vi "TLB Native Dynamic Events ver 0.11.vi"() -> ()   [LabVIEW 2018]
uses:
  Labview Training Phase 2/Enum Controls/States for Action Engine.ctl
  TLB Type Definitions/State Type Definitions, for 0.26g versions and later 2.ctl
  TLB Type Definitions/Intruction Type Definitions.ctl
  TLB Type Definitions/Encoder cluster.ctl
  Experimental VI's/Archived VI's/MOTOR CONTROL NO PID Type Def.ctl
  Underlying VI's/I2C Master VI/I2C MASTER Type Def.ctl
  TLB Type Definitions/PING CLUSTER.ctl
  <vilib>/Studica/Studica Toolkit/NavX/NavX.lvlib
  <vilib>/Studica/Studica Toolkit/Background/DIO Channel.ctl
  Underlying VI's/NavX VI/navX type def.ctl
  <vilib>/myRIO/Instrument Drivers/Utilities/Utilities.lvlib
  <vilib>/Studica/Studica Toolkit/Background/I2C Channel.ctl
  <vilib>/Studica/Studica Toolkit/NavX/TypeDefs/Flags/Z900_navX_Flags_CalibrationStatusTypeDef.ctl
  <vilib>/Studica/Studica Toolkit/NavX/TypeDefs/Flags/Z900_navX_Flags_OpStatusTypeDef.ctl
panel:
  out "Detect?":bool
  out "Status":T3 {"OP Status" items=["INITIALIZING", "SELFTEST_IN_PROGRESS", "ERROR", "IMU_AUTOCAL_IN_PROGRESS", "NORMAL"]; "Calibration Status" items=["IMU_CAL_STATE_MASK"=3, "IMU_CAL_STATE_INPROGRESS"=0, "IMU_CAL_STATE_ACCUMULATE"=1, "IMU_CAL_STATE_COMPLETE"=2]}
  out "NavX Readings":T4
  out "TASK ENABLE":bool
  out "Rising Edge":bool
  in  "Green LED":bool
  out "Task Selection":u8
  out "Object detected?":bool
  in  "Arduino Mode":T5=enum."Mode 0"
  out "Arduino Data":T6
  out "I2C Error":errorcluster
  out "Speed & distance":T7
  out "State Logic":T8=enum."Startup"
  out "elements":T9[](array[typedef])
  in  "STOP TASK":bool
  in  "OK Button":bool
  in  "STOP":bool
  out "error out":errorcluster
  out "Action Queue Items":i32
  out "State Logic Queue Items":i32
  out "Action Queues items":string[](array[string])=["Hardware reset", "Software reset", ""]
  out "Action State":string
  # "TLB FRAMEWORK STATUS"
  # "System Health Status Update"
  # "Test Programme written by Calvin Loke    Dated: 28 Aug 2019\nTest Programme revised by Dr Alex See   Dated 30 Aug 2019\n\nProgramme version:   TLB Native Dynamic Events ver 0.04b.vi"
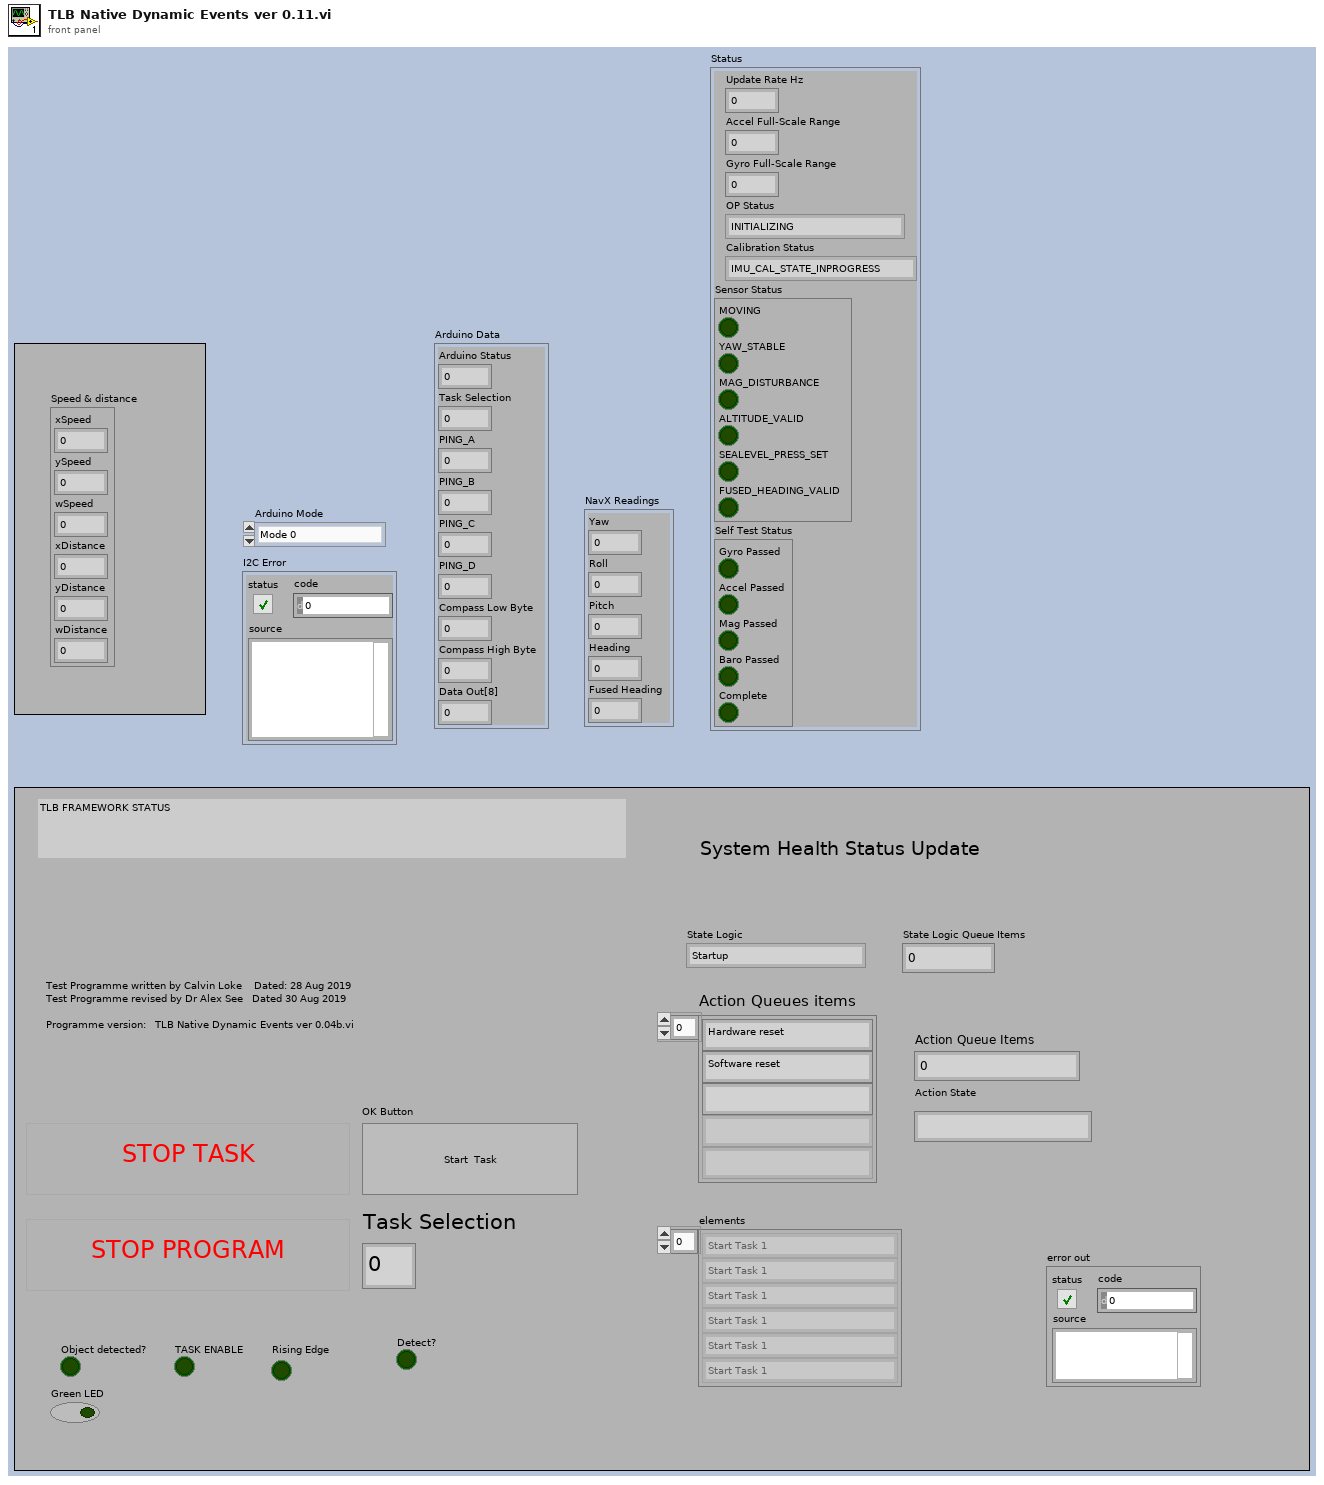
[diagram p1: front panel]
types:
  T1 = typedef "NavX.lvlib/Z900_navX_Flags_OpStatusTypeDef.ctl" = u8
  T2 = typedef "NavX.lvlib/Z900_navX_Flags_CalibrationStatusTypeDef.ctl" = u8
  T3 = cluster{"Update Rate Hz":u8, "Accel Full-Scale Range":u8, "Gyro Full-Scale Range":u16, "OP Status":T1, "Calibration Status":T2, "Sensor Status":cluster{"MOVING":bool, "YAW_STABLE":bool, "MAG_DISTURBANCE":bool, "ALTITUDE_VALID":bool, "SEALEVEL_PRESS_SET":bool, "FUSED_HEADING_VALID":bool}, "Self Test Status":cluster{"Gyro Passed":bool, "Accel Passed":bool, "Mag Passed":bool, "Baro Passed":bool, "Complete":bool}}
  T4 = cluster{"Yaw":dbl, "Roll":dbl, "Pitch":dbl, "Heading":dbl, "Fused Heading":dbl}
  T5 = typedef "I2C MASTER Type Def.ctl" = enum16{"Last State", "Mode 0", "Mode 1", "Mode 2", "Mode 3", "Mode 4", "Mode 5", "Mode 6", "Mode 7", "Mode 8", "Mode 9", "Mode 10"}
  T6 = cluster{"Arduino Status":u8, "Task Selection":u8, "PING_A":u8, "PING_B":u8, "PING_C":u8, "PING_D":u8, "Compass Low Byte":u8, "Compass High Byte":u8, "Data Out[8]":u8}
  T7 = cluster{"xSpeed":dbl, "ySpeed":dbl, "wSpeed":dbl, "xDistance":dbl, "yDistance":dbl, "wDistance":dbl}
  T8 = typedef "State Type Definitions, for 0.26g versions and later 2.ctl" = enum16{"None", "Startup", "Move to Angle", "True Stop", "Idle", "Shutdown", "Task 1A", "Task 1B", "Task 2:Raise Arm", "Task 2:Sensor Mode", "Task 2:Reverse Mode", "Task 3", "Task 4_A", "Task 4_B", "Task 4_C", "Task 4_D", "Task 5A", "Task 5B", "Task 5C", "Task 5D", "Task 5E: POSITION ARM", "Task 5F: ARM GRAB HEIGHT", "Task 5G: CLOSE CLAW", "Task 5H: RAISE ARM", "Task 6_A", "Task 6_B", "Task 7", "Task 8A: RAISE ARM", "Task 8B: MOVE TO BOX", "Task 8C: CAM BURST", "Task 8D: PROCESS IMAGE", "Task 8E: ROBOT ADJUST", "Task 8F: CAM BURST 2", "Task 8G: PROCESS IMAGE 2", "Task 8H: ARM ADJUST", "Task 8I: ARM GRAB HEIGHT", "Task 8J: CLOSE CLAW", "Task 8K: RAISE MY SWORD", "Task 9A: Raise Arm", "Task 9B: Rotate to Angle", "Task 9C: Detect Box", "Task 9D: MOVE FORWARD", "Task 9E: MOVE LEFT", "Task 9F: SCAN BOX", "Task 9G: MOVE RIGHT", "Task 9H: SCAN BOX 2", "Task 9I: ROTATE 90 CW", "Task 9J: FORWARD", "Task 9K: RAM WALL", "Task 9L: MOVE RIGHT", "Task 9M: SCAN BOX 3", "Task 9M: MOVE RIGHT", "Task 9N: SCAN BOX 4", "PENIS", "PENIS 2", "PENIS 3", "Task 9R: PROCESS COLOUR", "Task A1: Task 9 Open cam", "Task A2: Task 9 Move Arm", "Task A3: Task 9 Set Timer", "Task A4: Tasl 9 Capture images", "Task A5: Task 9 Close camera", "Task A6: Process Colour", "Task A7: Dispose Camera Buffer"}
  T9 = typedef "Intruction Type Definitions.ctl" = enum16{"None", "Start Task 1", "Start Task 2", "Start Task 3", "Start Task 4", "Start Task 5", "Start Task 6", "Start Task 7", "Start Task 8 - BALL", "Start Task 8 - Gel", "Start Task 8 - Pipe", "Start Task 8 - Soap", "Start Task 9", "Start Task A", "Start Task B", "Exit"}
  T10 = typedef "States for Action Engine.ctl" = enum16{"Initialize", "Write", "Read"}
  T11 = typedef "DIO Channel.ctl" = enum16{"Not Connected", "A/DIO1", "A/DIO2", "A/DIO3", "A/DIO4", "A/DIO5", "A/DIO6", "A/DIO7", "A/DIO13", "B/DIO1", "B/DIO2", "B/DIO3", "B/DIO4", "B/DIO5", "B/DIO6", "B/DIO7", "B/DIO13", "C/DIO0", "C/DIO1", "C/DIO2", "C/DIO3", "C/DIO4", "C/DIO5", "C/DIO6", "C/DIO7"}
  T12 = typedef "PING CLUSTER.ctl" = cluster{"PING_A":u8, "PING_B":u8, "PING_C":u8, "PING_D":u8}
  T13 = typedef "Encoder cluster.ctl" = cluster{"xDistance":dbl, "yDistance":dbl, "wDistance":dbl}
  T14 = typedef "I2C Channel.ctl" = enum16{"Not Connected", "A", "B"}
  T15 = typedef "navX type def.ctl" = enum16{"Get i2C reference", "Read Values", "Zero Yaw"}
  T16 = typedef "State Type Definitions.ctl" = enum16{"None", "Startup", "Move to Angle", "True Stop", "Idle", "Shutdown", "Task 1", "Task 2:Raise Arm", "Task 2:Sensor Mode", "Task 2:Reverse Mode", "Task 3", "Task 4_A", "Task 4_B", "Task 4_C", "Task 4_D", "Task 5A: ARM CAM HEIGHT", "Task 5B: MOVE TO BOX", "Task 5C: CAM BURST", "Task 5D: PROCESS IMAGE", "Task 5E: POSITION ARM", "Task 5F: ARM GRAB HEIGHT", "Task 5G: CLOSE CLAW", "Task 5H: RAISE ARM", "Task 6_A", "Task 6_B", "Task 7", "Task 8A: RAISE ARM", "Task 8B: MOVE TO BOX", "Task 8C: CAM BURST", "Task 8D: PROCESS IMAGE", "Task 8E: ROBOT ADJUST", "Task 8F: CAM BURST 2", "Task 8G: PROCESS IMAGE 2", "Task 8H: ARM ADJUST", "Task 8I: ARM GRAB HEIGHT", "Task 8J: CLOSE CLAW", "Task 8K: RAISE MY SWORD", "Task 9A: Raise Arm", "Task 9B: Rotate to Angle", "Task 9C: Detect Box", "Task 9D: MOVE FORWARD", "Task 9E: MOVE LEFT", "Task 9F: SCAN IMAGE", "Task 9G: PROCESS COLOUR", "Task 9H: MOVE RIGHT", "Task 9I: SCAN IMAGE", "Task 9J: PROCESS COLOUR", "Task 9K: ROTATE 90 CW", "Task 9L: MOVE FORWARD", "Task 9M: MOVE RIGHT", "Task 9N: SCAN IMAGE", "Task 9O: PROCESS COLOUR", "Task 9P: MOVE RIGHT", "Task 9Q: SCAN IMAGE", "Task 9R: PROCESS COLOUR"}
  T17 = typedef "State Type Definitions.ctl" = enum16{"None", "Startup", "Move to Angle", "True Stop", "Idle", "Shutdown", "Task 1", "Task 2", "Task 3", "Task 4_A", "Task 4_B", "Task 4_C", "Task 5", "Task 6", "Task 7", "Task 8", "Task 9", "Task A", "Task B"}
  T18 = typedef "MOTOR CONTROL NO PID Type Def.ctl" = enum16{"Init", "Front Back", "Left Right", "Rotate", "Stop", "Latch"}
  T19 = cluster{"DIO Channel":T11, "FPGA VI Reference Out":refnum<k20>}
  T20 = cluster{"I2C Ref Out":cluster{"I2C Channel":T14, "FPGA VI Reference Out":refnum<k20>}, "Connected":bool, "Slave Address (7-bit)":u8, "Registry":u8[]}
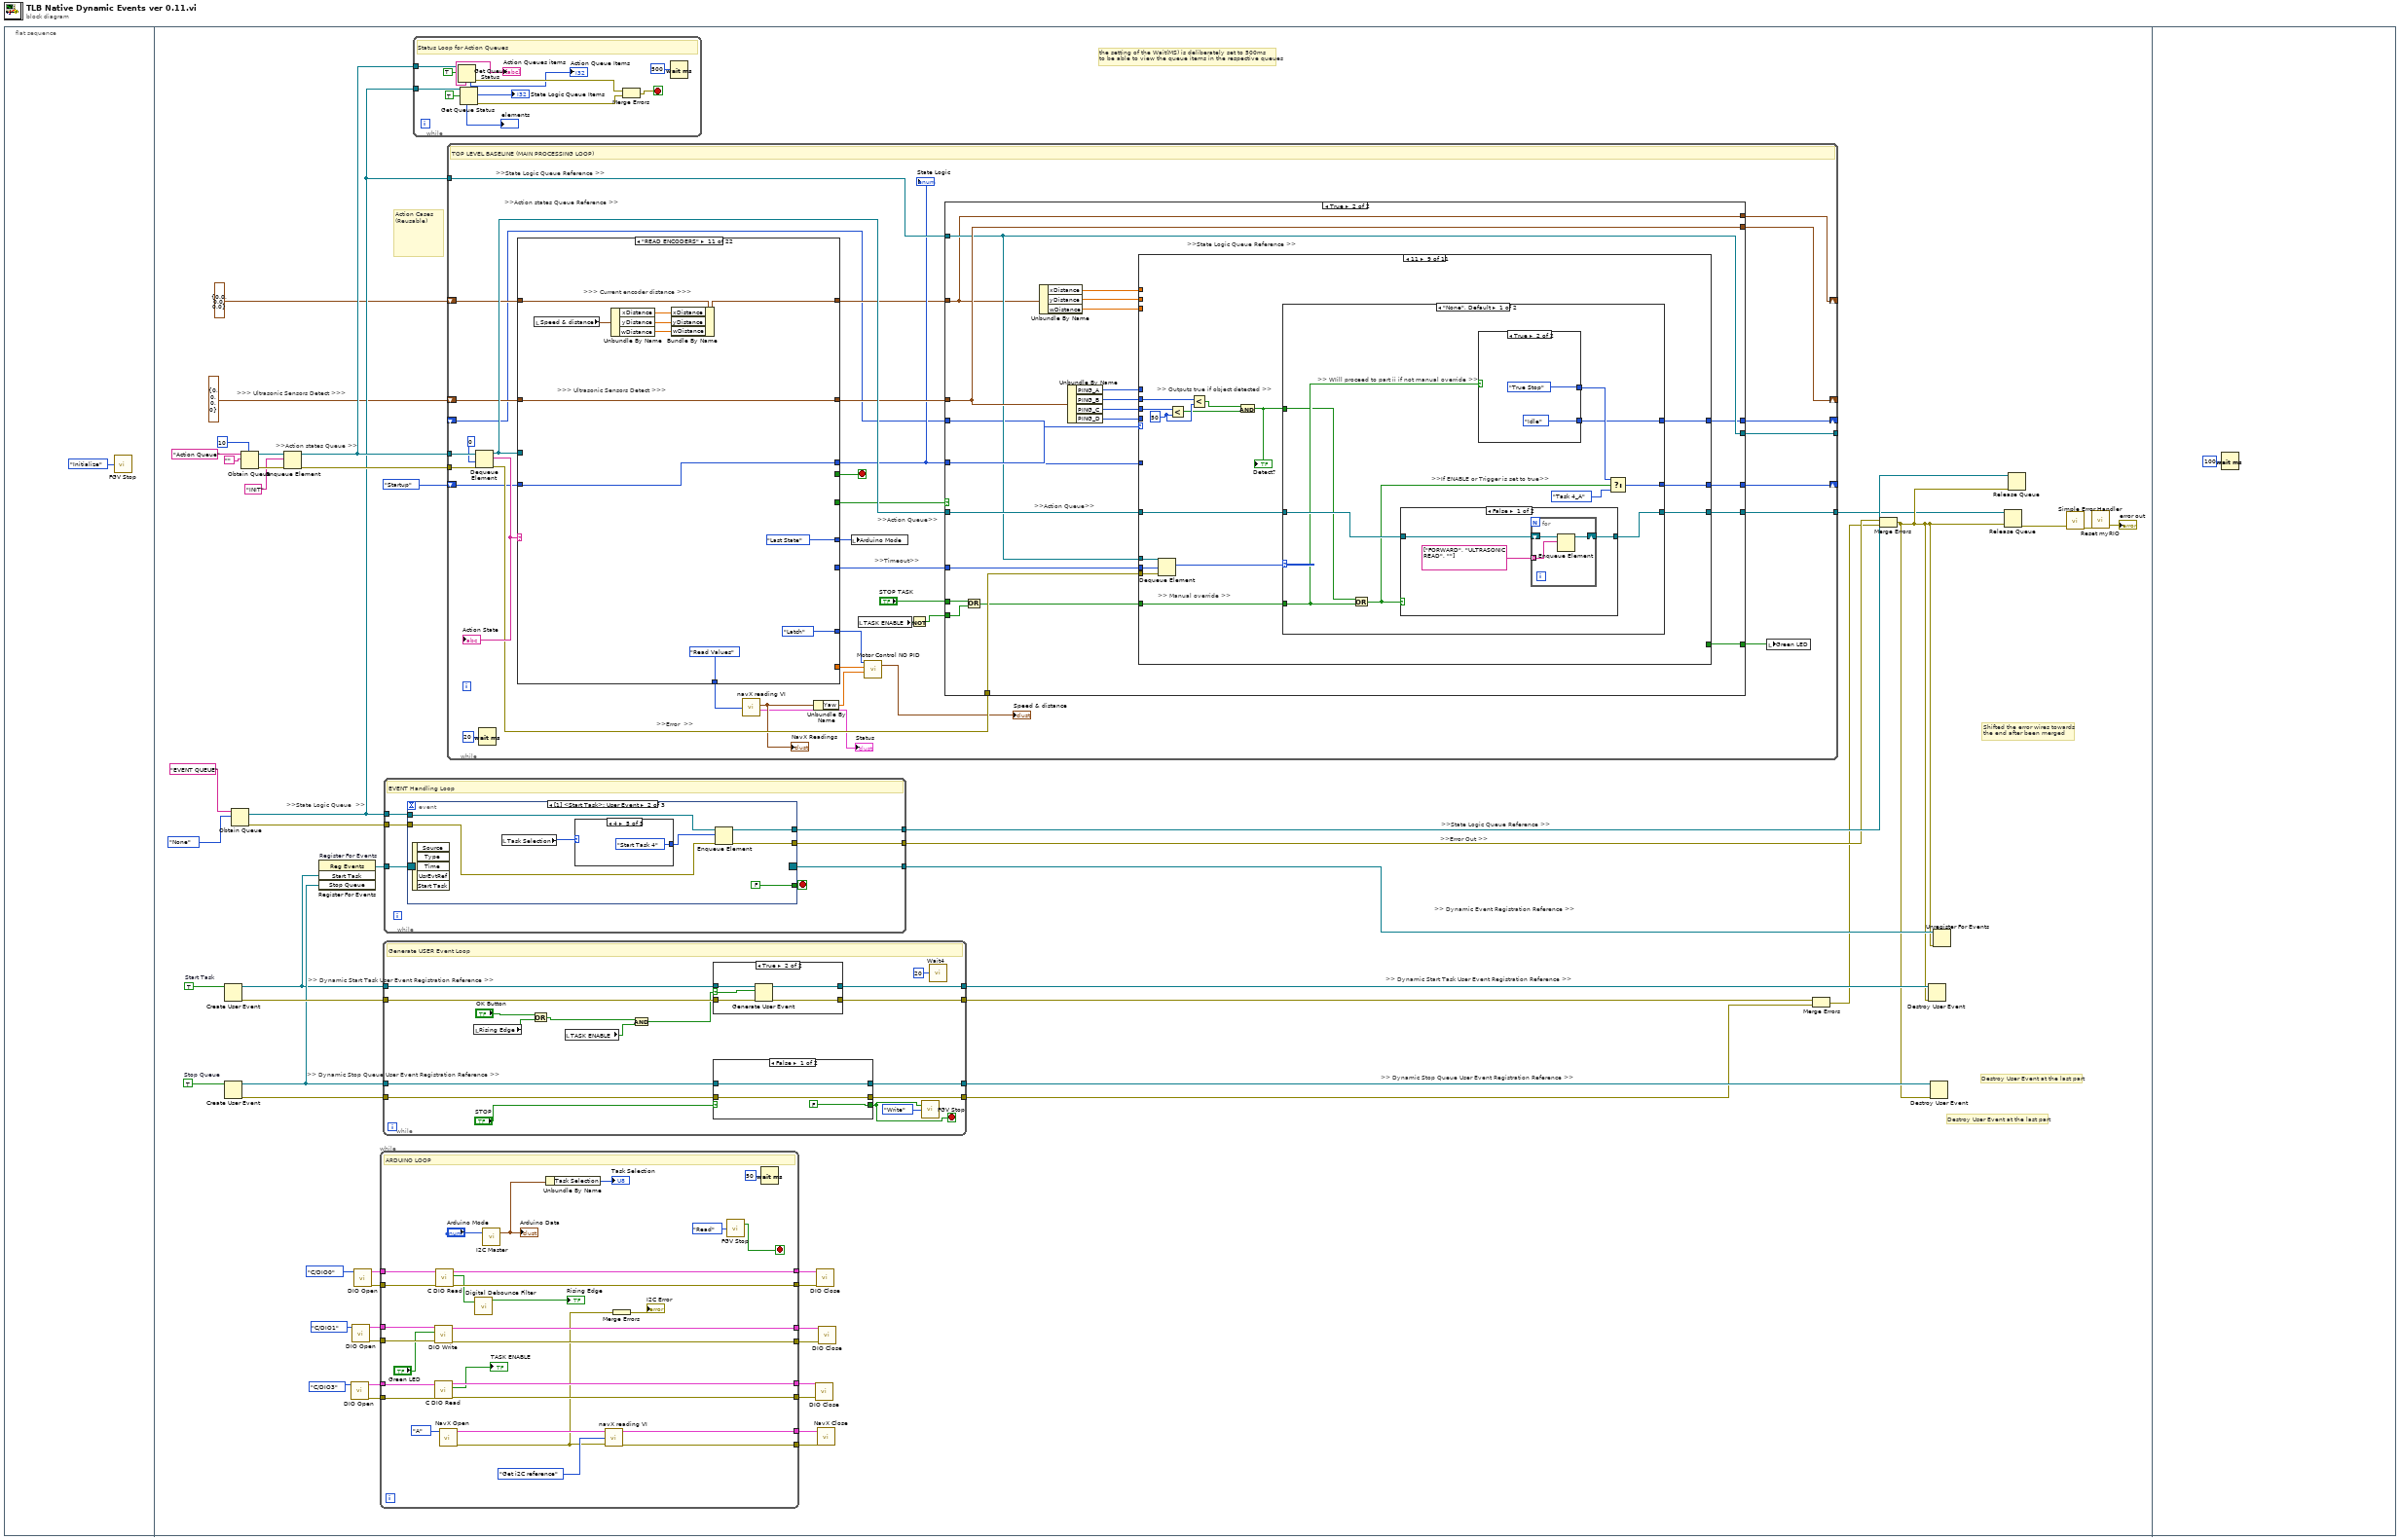
[diagram p0: block diagram]
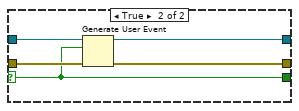
[diagram p2: hidden frame]
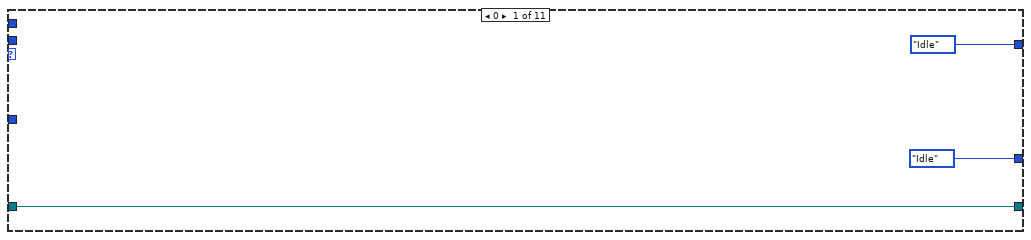
[diagram p5: hidden frame]
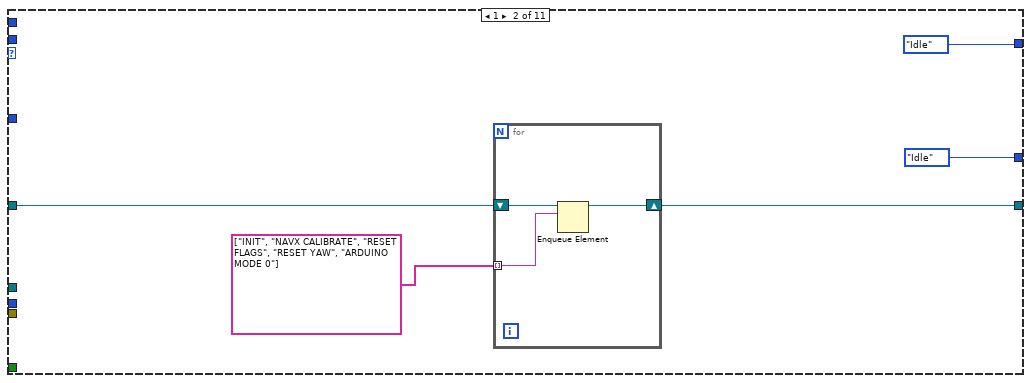
[diagram p6: hidden frame]
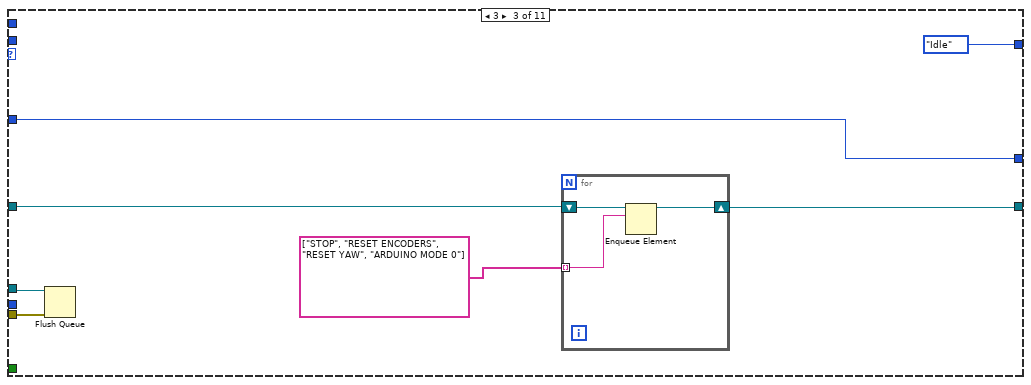
[diagram p7: hidden frame]
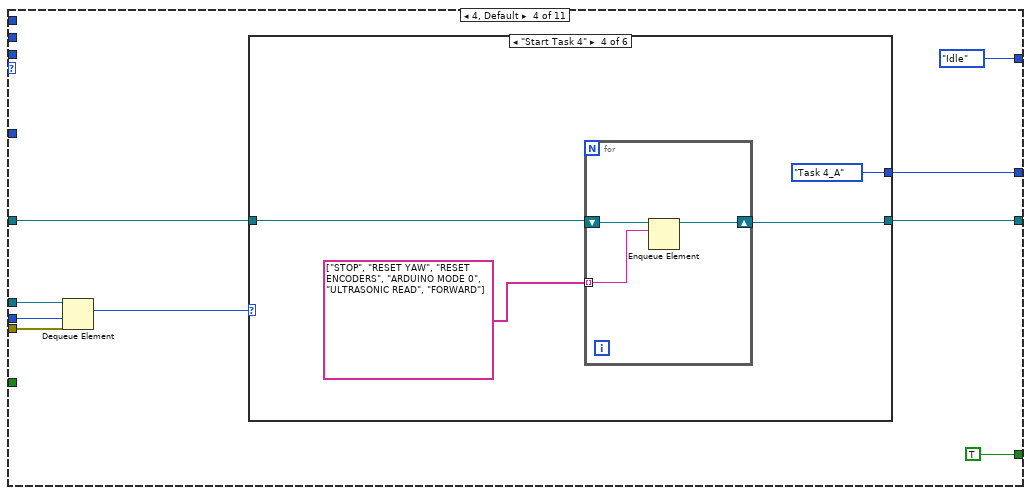
[diagram p8: hidden frame]
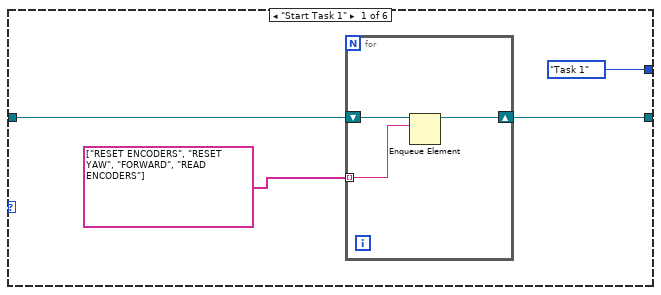
[diagram p9: hidden frame]
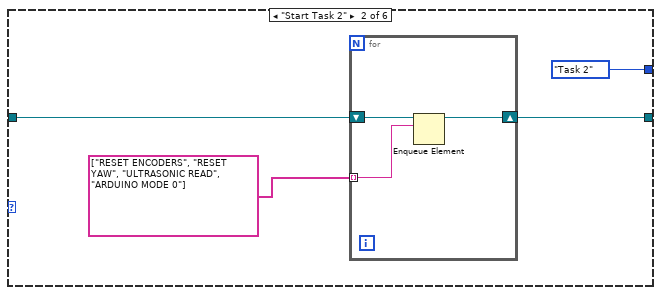
[diagram p10: hidden frame]
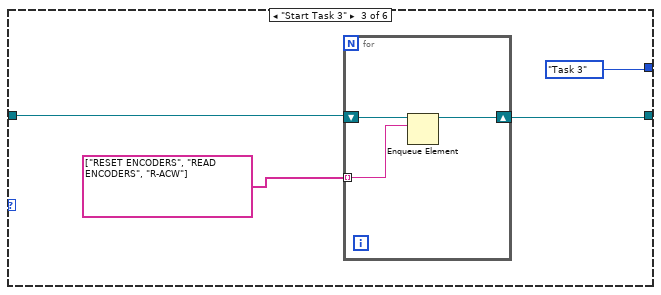
[diagram p11: hidden frame]
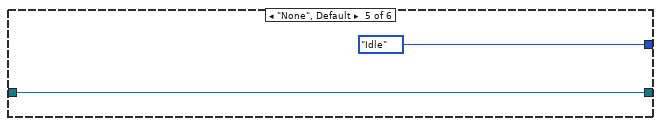
[diagram p12: hidden frame]
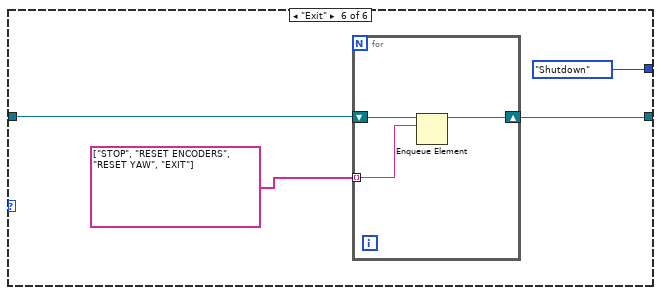
[diagram p13: hidden frame]
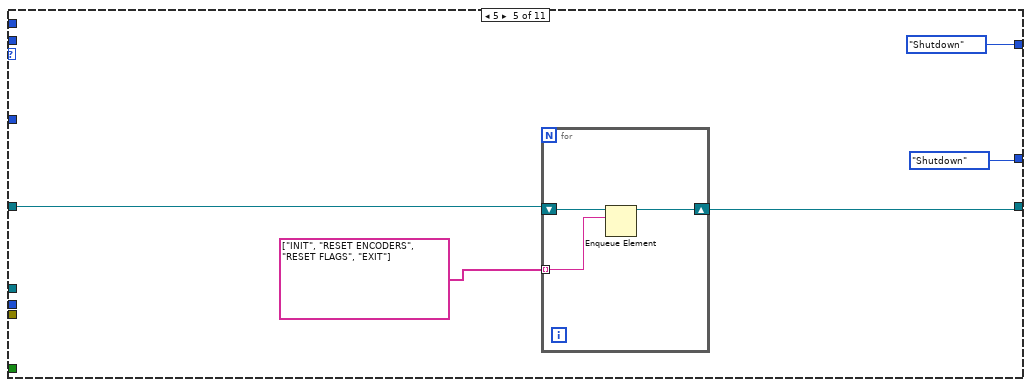
[diagram p14: hidden frame]
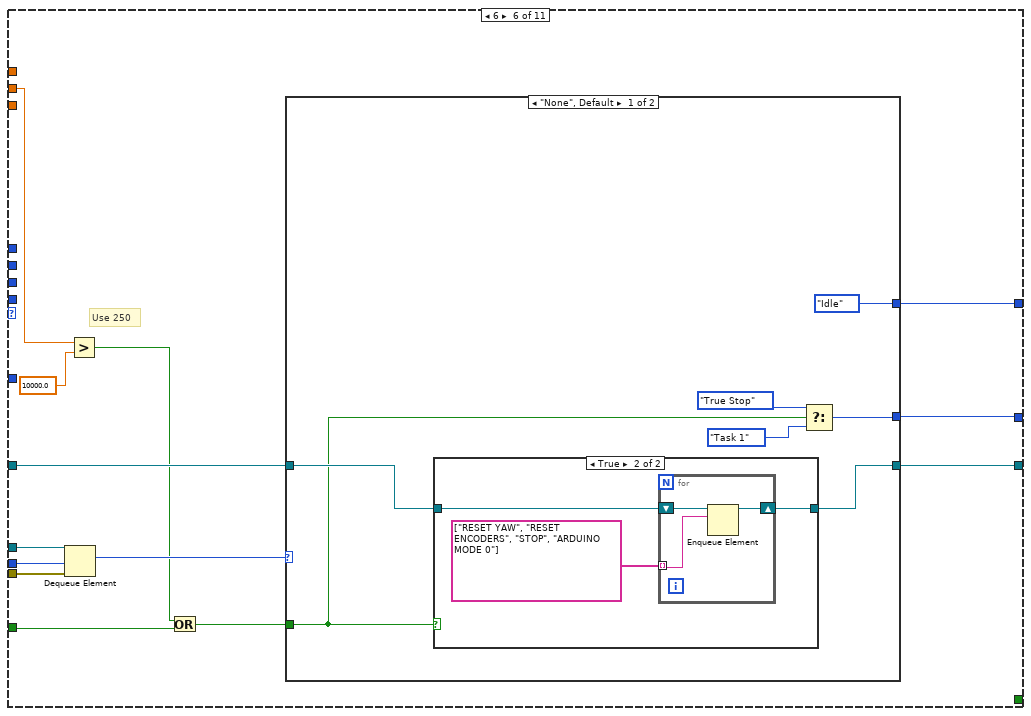
[diagram p15: hidden frame]
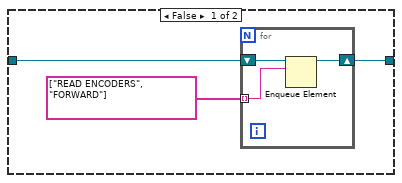
[diagram p16: hidden frame]
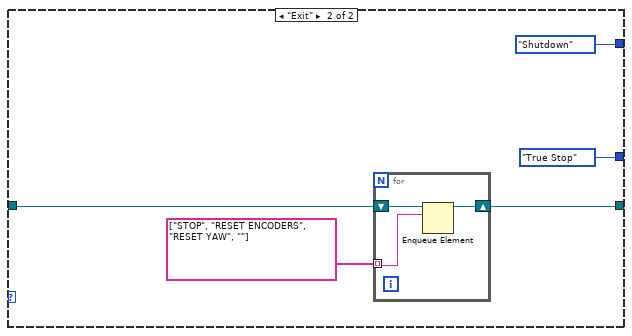
[diagram p17: hidden frame]
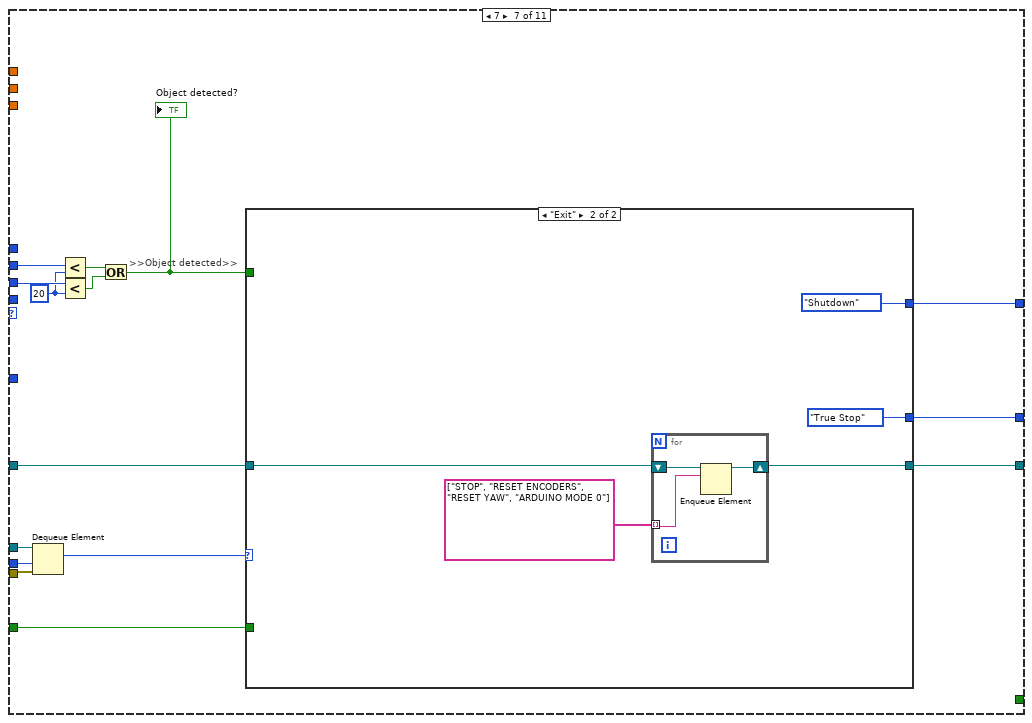
[diagram p18: hidden frame]
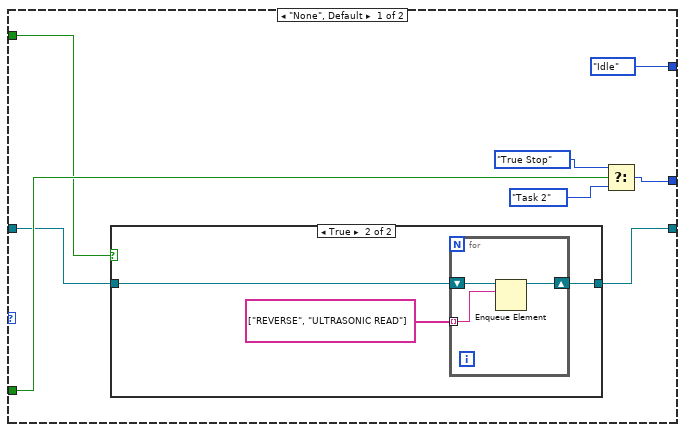
[diagram p19: hidden frame]
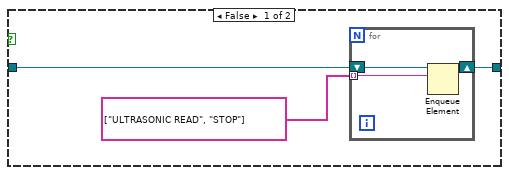
[diagram p20: hidden frame]
diagram:
  n1 = flat-sequence {
    frame #0 {
      n2 = call "FGV Stop.vi"("Init/Read/Write State"=States_for_Action_Engine."Initialize") -> ()  [unwired: 2 in, 2 out]
    }
    frame #1 {
      w53 = TRUE  # Stop Queue
      w52 = TRUE  # Start Task
      # ">>> Ultrasonic Sensors Detect >>>"
      # "the setting of the Wait(MS) is deliberately set to 500ms\nto be able to view the queue items in the respective queues"
      # "Action Cases\n(Reusable)"
      # ">>Error Out >>"
      # ">> Dynamic Stop Queue User Event Registration Reference >>"
      # ">> Dynamic Start Task User Event Registration Reference >>"
      # ">> Dynamic Stop Queue User Event Registration Reference >>"
      # ">> Dynamic Start Task User Event Registration Reference >>"
      # ">> Dynamic Event Registration Reference >>"
      # ">>Action states Queue >>"
      # ">>State Logic Queue  >>"
      # ">>State Logic Queue Reference >>"
      # "Destroy User Event at the last part"
      # "Destroy User Event at the last part"
      # "Shifted the error wires towards\nthe end after been merged"
      n3 = Create User Event(user event datatype=w52) -> (user event=w44:refnum<user-event>, error out=w49:errorcluster)  [unwired: 1 in]
      n4 = Create User Event(user event datatype=w53) -> (user event=w45:refnum<user-event>, error out=w48:errorcluster)  [unwired: 1 in]
      n5 = Obtain Queue(name (unnamed)="EVENT QUEUE", element data type=Intruction_Type_Definitions."None" ("Enum")) -> (queue out=w30:refnum<queue>, error out=w36:errorcluster)  [unwired: 3 in, 1 out]
      n6 = Obtain Queue(max queue size (-1, unlimited)=10, name (unnamed)="Action Queue", element data type="") -> (queue out=w39:refnum<queue>, error out=w35:errorcluster)  [unwired: 2 in, 1 out]
      n7 = Enqueue Element(queue=w39, element="INIT", error in (no error)=w35) -> (queue out=w31:refnum<queue>, error out=w34:errorcluster)  [unwired: 1 in, 1 out]
      n8 = register-events "Register For Events"(w44, w45) -> (reference out=w43:refnum<event-registration>)  [unwired: 2 in, 1 out]
      n9 = call <vilib>:"DIO Open.vi"("DIO Channel"=DIO_Channel."C/DIO3") -> ("error out"=w8:errorcluster, "DIO Info Out"=w9:T19)  [unwired: 9 in]
      n10 = call <vilib>:"DIO Open.vi"("DIO Channel"=DIO_Channel."C/DIO1") -> ("error out"=w13:errorcluster, "DIO Info Out"=w15:T19)  [unwired: 9 in]
      n11 = call <vilib>:"DIO Open.vi"("DIO Channel"=DIO_Channel."C/DIO0") -> ("error out"=w18:errorcluster, "DIO Info Out"=w21:T19)  [unwired: 9 in]
      n12 = while {
        tunnel: w21 -> [w77]
        tunnel: [w76] -> w19
        tunnel: w18 -> [w75]
        tunnel: [w74] -> w17
        tunnel: w15 -> [w69]
        tunnel: [w68] -> w14
        tunnel: w13 -> [w67]
        tunnel: [w66] -> w12
        tunnel: [w64] -> w10
        tunnel: w9 -> [w63]
        tunnel: w8 -> [w62]
        tunnel: [w61] -> w7
        tunnel: [w58] -> w6
        tunnel: [w57] -> w5
        stop <- w81 stop-if-true
        # "ARDUINO LOOP"
        n13 = call <vilib>:"DIO Write.vi"("error in (no error)"=w67, "Input"="Green LED", "DIO Info In"=w69) -> ("error out"=w66:errorcluster, "DIO Info Out"=w68:T19)  [unwired: 7 in]
        n14 = call <vilib>:"C DIO Read.vi"("error in (no error)"=w62, "DIO Info In in"=w63) -> ("error out"=w61:errorcluster, "IN"=→"TASK ENABLE":bool, "DIO Info In out"=w64:T19)  [unwired: 7 in]
        n15 = call <vilib>:"C DIO Read.vi"("error in (no error)"=w75, "DIO Info In in"=w77) -> ("error out"=w74:errorcluster, "IN"=w72:bool, "DIO Info In out"=w76:T19)  [unwired: 7 in]
        n16 = call <vilib>:"NavX Open.vi"("I2C Channel"=I2C_Channel."A") -> ("error out"=w55:errorcluster, "NavX Info"=w59:T20)  [unwired: 9 in]
        n17 = call "Digital Debounce Filter.vi"("Boolean input"=w72) -> ("Rising Edge"=→"Rising Edge":bool)  [unwired: 1 in, 2 out]
        n18 = call "I2C Master.vi"("Arduino Mode"="Arduino Mode") -> ("Arduino Data"=w70:T6)  [unwired: 1 in, 1 out]
        "Arduino Data" <- w70
        n19 = Unbundle By Name(w70) -> ("Task Selection"=→"Task Selection":u8)
        n20 = call "navX reading VI.vi"("NavX Info In"=w59, "Mode"=navX_type_def."Get i2C reference", "error in (no error)"=w55) -> ("NavX Info Out"=w58:T20, "Error Out"=w57:errorcluster)  [unwired: 2 out]
        n21 = Merge Errors(w55) -> (→"I2C Error":errorcluster)
        n22 = call "FGV Stop.vi"("Init/Read/Write State"=States_for_Action_Engine."Read") -> ("Output node"=w81:bool)  [unwired: 2 in, 1 out]
        n23 = Wait (ms)(milliseconds to wait=u32 50) -> ()  [unwired: 1 out]
      }
      n24 = while {
        tunnel: w44 -> [w111]
        tunnel: w45 -> [w110]
        tunnel: [w109] -> w51
        tunnel: [w108] -> w50
        tunnel: w49 -> [w107]
        tunnel: [w106] -> w47
        tunnel: w48 -> [w105]
        tunnel: [w104] -> w46
        stop <- w102 stop-if-true
        # "Generate USER Event Loop"
        n25 = local read "Rising Edge"() -> (w98:bool)
        n26 = Or(x="OK Button", y=w98) -> (x .or. y?=w97:bool)
        n27 = local read "TASK ENABLE"() -> (w96:bool)
        n28 = And(x=w97, y=w96) -> (x .and. y?=w95:bool)
        n29 = case shown="True" w95 {
          selector: w95 -> [_ w122]
          tunnel: w111 -> [w121 w126]
          tunnel: [w121 w125] -> w108
          tunnel: w107 -> [w120 w124]
          tunnel: [w120 w123] -> w106
          frame False {
          }
          frame True {
            n30 = Generate User Event(user event=w126, event data cluster=w122, error in=w124) -> (user event out=w125:refnum<user-event>, error out=w123:errorcluster)  [unwired: 1 in]
          }
        }
        n31 = case shown="False" "STOP" {
          selector: "STOP" -> [_ w115]
          tunnel: w110 -> [w114 w119]
          tunnel: [w114 w118] -> w109
          tunnel: w105 -> [w113 w117]
          tunnel: [w113 w116] -> w104
          tunnel: [FALSE w115] -> w102
          frame False {
          }
          frame True {
            n32 = Generate User Event(user event=w119, event data cluster=w115, error in=w117) -> (user event out=w118:refnum<user-event>, error out=w116:errorcluster)  [unwired: 1 in]
          }
        }
        n33 = call "FGV Stop.vi"("Init/Read/Write State"=States_for_Action_Engine."Write", "Input Node"=w102) -> ()  [unwired: 1 in, 2 out]
        n34 = call "Wait4"("Count(uSec)"=u32 20) -> ()  [unwired: 1 out]
      }
      n35 = while {
        tunnel: w43 -> [w684]
        tunnel: [w683] -> w42
        tunnel: w30 -> [w681]
        tunnel: [w680] -> w41
        tunnel: w36 -> [w679]
        tunnel: [w678] -> w33
        stop <- w682 stop-if-true
        # "EVENT Handling Loop"
        n36 = event shown="[1] <Start Task>: User Event" {
          selector: w684 -> [_ _ _]
          dyn-events: [_ _ _] -> w683
          timeout: _ -> [_ _ _]
          tunnel: [FALSE FALSE w708] -> w682
          tunnel: w681 -> [w689 w696 w706]
          tunnel: [w688 w695 w707] -> w680
          tunnel: w679 -> [w687 w694 w705]
          tunnel: [w686 w693 w704] -> w678
          event Timeout {
            n37 = event-data() -> ()  [unwired: 1 in, 3 out]
            n38 = Enqueue Element(queue=w689, element=Intruction_Type_Definitions."None" ("Enum"), error in (no error)=w687) -> (queue out=w688:refnum<queue>, error out=w686:errorcluster)  [unwired: 1 in, 1 out]
          }
          event User Event {
            n39 = event-data() -> ()  [unwired: 1 in, 5 out]
            n40 = local read "Task Selection"() -> (w691:u8)
            n41 = case shown="4" w691 {
              tunnel: [Intruction_Type_Definitions."None" ("Enum") Intruction_Type_Definitions."Start Task 1" ("Enum") Intruction_Type_Definitions."Start Task 2" ("Enum") Intruction_Type_Definitions."Start Task 3" ("Enum") Intruction_Type_Definitions."Start Task 4" ("Enum")] -> w692
              frame 0, Default {
              }
              frame 1 {
              }
              frame 2 {
              }
              frame 3 {
              }
              frame 4 {
              }
            }
            n42 = Enqueue Element(queue=w696, element=w692, error in (no error)=w694) -> (queue out=w695:refnum<queue>, error out=w693:errorcluster)  [unwired: 1 in, 1 out]
          }
          event User Event {
            n43 = event-data() -> ("Stop Queue"=w708:bool)  [unwired: 1 in, 4 out]
            n44 = Enqueue Element At Opposite End(queue=w706, element=Intruction_Type_Definitions."Exit" ("Enum"), error in (no error)=w705) -> (queue out=w707:refnum<queue>, error out=w704:errorcluster)  [unwired: 1 in, 1 out]
          }
        }
      }
      n45 = while {
        tunnel: w31 -> [w92]
        tunnel: w30 -> [w89]
        stop <- w86 stop-if-true
        # "Status Loop for Action Queues"
        n46 = Get Queue Status(queue=w92, return elements? (F)=TRUE) -> (error out=w88:errorcluster, # elements in queue=→"Action Queue Items":i32, elements=→"Action Queues items":string[])  [unwired: 1 in, 5 out]
        n47 = Get Queue Status(queue=w89, return elements? (F)=TRUE) -> (# pending remove=→"State Logic Queue Items":i32, error out=w87:errorcluster, elements=→"elements":T9[])  [unwired: 1 in, 5 out]
        n48 = Merge Errors(w88, w87) -> (w86:errorcluster)
        n49 = Wait (ms)(milliseconds to wait=u32 500) -> ()  [unwired: 1 out]
      }
      n50 = while {
        tunnel: w30 -> [w150]
        tunnel: w31 -> [w162]
        tunnel: w34 -> [w160]
        tunnel: [w159] -> _
        tunnel: [w158] -> w24
        shift-right: [w151] -> _
        shift-left: T12 {"PING_A"=0, "PING_B"=0, "PING_C"=0, "PING_D"=0} -> [w153]
        shift-right: [w144] -> _
        shift-left: State_Type_Definitions,_for_0.26g_versions_and_later_2."Startup" ("Enum") -> [w147]
        shift-right: [w140] -> _
        shift-left: T13 {"xDistance"=0.0, "yDistance"=0.0, "wDistance"=0.0} -> [w142]
        shift-right: [w133] -> _
        shift-left: _ -> [w132]
        stop <- w149 stop-if-true
        # ">>Error  >>"
        # ">>Action Queue>>"
        # ">>Timeout>>"
        # ">>Action states Queue Reference >>"
        # ">>State Logic Queue Reference >>"
        # "TOP LEVEL BASELINE (MAIN PROCESSING LOOP)"
        n51 = Dequeue Element(queue=w162, timeout in ms (-1)=0, error in (no error)=w160) -> (queue out=w154:refnum<queue>, element=w161:string, error out=w155:errorcluster)  [unwired: 1 out]
        "Action State" <- w161
        n52 = Wait (ms)(milliseconds to wait=u32 20) -> ()  [unwired: 1 out]
        n53 = case shown="\"READ ENCODERS\"" w161 {
          tunnel: [_ _ _ _ _ _ _ _ _ _ _ _ _ _ _ _ 0 w651 _ _ _ _] -> w157
          tunnel: w154 -> [_ _ _ _ _ _ _ _ _ _ _ _ _ _ _ _ _ _ _ _ _ _]
          tunnel: w153 -> [w539 w544 w551 w557 w563 w568 w575 w582 w588 w591 w603 w614 w618 w628 w632 w636 w644 w652 w657 w662 w669 w677]
          tunnel: [w539 w544 w551 w557 w563 w568 w575 w582 w588 w591 w603 w615 w618 w629 w632 w636 w644 w652 w657 w662 w668 w677] -> w152
          tunnel: [TRUE TRUE _ _ _ _ _ _ _ _ _ _ _ _ _ _ _ _ _ _ _ _] -> w149
          tunnel: w147 -> [w537 w542 w550 w556 w562 w567 w574 w581 w587 w590 w602 w613 w617 w627 w631 w635 w641 w649 w656 w661 w667 w676]
          tunnel: [_ _ _ _ _ _ _ _ _ _ _ _ _ _ _ _ _ TRUE _ _ _ _] -> w146
          tunnel: [w537 w542 w550 w556 w562 w567 w574 w581 w587 w590 w602 w613 w617 w627 w631 w635 w641 w649 w656 w661 w667 w676] -> w145
          tunnel: w142 -> [w536 w541 w549 w555 w561 w566 w573 w580 w586 w592 w601 w612 w619 w626 w633 w637 w640 w648 w658 w663 w666 w675]
          tunnel: [w536 w541 w549 w555 w561 w566 w573 w580 w586 w592 w600 w612 w619 w625 w633 w637 w640 w648 w658 w663 w666 w675] -> w141
          tunnel: [_ _ 0.4 ("Speed") -0.3 ("Speed") 0.19999999999999998 ("Speed") -0.2 ("Speed") _ 0.3 ("Speed") -0.5 ("Speed") _ _ _ _ 0.0 ("Speed") _ _ _ _ _ _ _ _] -> w139
          tunnel: [_ _ MOTOR_CONTROL_NO_PID_Type_Def."Front Back" ("Direction") _ MOTOR_CONTROL_NO_PID_Type_Def."Rotate" ("Direction") _ MOTOR_CONTROL_NO_PID_Type_Def."Stop" ("Direction") MOTOR_CONTROL_NO_PID_Type_Def."Left Right" ("Direction") MOTOR_CONTROL_NO_PID_Type_Def."Front Back" ("Direction") _ MOTOR_CONTROL_NO_PID_Type_Def."Latch" ("Direction") MOTOR_CONTROL_NO_PID_Type_Def."Latch" ("Direction") _ _ _ _ _ MOTOR_CONTROL_NO_PID_Type_Def."Latch" ("Direction") _ MOTOR_CONTROL_NO_PID_Type_Def."Init" ("Direction") _ MOTOR_CONTROL_NO_PID_Type_Def."Init" ("Direction")] -> w137
          tunnel: [I2C_MASTER_Type_Def."Last State" ("Arduino Mode") I2C_MASTER_Type_Def."Last State" ("Arduino Mode") I2C_MASTER_Type_Def."Last State" ("Arduino Mode") I2C_MASTER_Type_Def."Last State" ("Arduino Mode") I2C_MASTER_Type_Def."Last State" ("Arduino Mode") I2C_MASTER_Type_Def."Last State" ("Arduino Mode") I2C_MASTER_Type_Def."Last State" ("Arduino Mode") I2C_MASTER_Type_Def."Last State" ("Arduino Mode") I2C_MASTER_Type_Def."Last State" ("Arduino Mode") I2C_MASTER_Type_Def."Last State" ("Arduino Mode") I2C_MASTER_Type_Def."Last State" ("Arduino Mode") I2C_MASTER_Type_Def."Mode 0" ("Arduino Mode") I2C_MASTER_Type_Def."Last State" ("Arduino Mode") I2C_MASTER_Type_Def."Last State" ("Arduino Mode") I2C_MASTER_Type_Def."Mode 0" ("Arduino Mode") I2C_MASTER_Type_Def."Mode 1" ("Arduino Mode") I2C_MASTER_Type_Def."Last State" ("Arduino Mode") I2C_MASTER_Type_Def."Last State" ("Arduino Mode") I2C_MASTER_Type_Def."Last State" ("Arduino Mode") I2C_MASTER_Type_Def."Last State" ("Arduino Mode") I2C_MASTER_Type_Def."Last State" ("Arduino Mode") I2C_MASTER_Type_Def."Last State" ("Arduino Mode")] -> w136
          tunnel: [_ _ navX_type_def."Read Values" ("Mode") navX_type_def."Read Values" ("Mode") _ _ navX_type_def."Read Values" ("Mode") navX_type_def."Read Values" ("Mode") _ _ navX_type_def."Read Values" ("Mode") navX_type_def."Read Values" ("Mode") _ navX_type_def."Zero Yaw" ("Mode") _ _ navX_type_def."Zero Yaw" ("Mode") navX_type_def."Read Values" ("Mode") _ _ _ navX_type_def."Zero Yaw" ("Mode")] -> w130
          frame "Exit" {
          }
          frame "----Movement States----" {
          }
          frame "FORWARD" {
          }
          frame "LEFT" {
          }
          frame "R-ACW" {
          }
          frame "R-CW" {
          }
          frame "STOP" {
            n54 = Wait (ms)(milliseconds to wait=u32 200) -> ()  [unwired: 1 out]
          }
          frame "RIGHT" {
          }
          frame "REVERSE" {
          }
          frame "----SENSOR READING---- " {
          }
          frame "READ ENCODERS" {
            # ">>> Current encoder distance >>>"
            # ">>> Ultrasonic Sensors Detect >>>"
            n55 = local read "Speed & distance"() -> (w599:T7)
            n56 = Unbundle By Name(w599) -> ("xDistance"=w598:dbl, "yDistance"=w597:dbl, "wDistance"=w596:dbl)
            n57 = Bundle By Name(cluster=w601, "xDistance"=w598, "yDistance"=w597, "wDistance"=w596) -> (w600:T13)
          }
          frame "ULTRASONIC READ" {
            # "Object detection"
            n58 = local read "Arduino Data"() -> (w610:T6)
            n59 = Unbundle By Name(w610) -> ("PING_A"=w609:u8, "PING_B"=w608:u8, "PING_C"=w607:u8, "PING_D"=w606:u8)
            n60 = Bundle By Name(cluster=w614, "PING_A"=w609, "PING_B"=w608, "PING_C"=w607, "PING_D"=w606) -> (w615:T12)
          }
          frame "----SYSTEM MODES----" {
          }
          frame "INIT" {
            w622 = 0
            w624 = 0.0
            # ">>State Logic  >>"
            n61 = Bundle By Name(cluster=w628, "PING_A"=w622, "PING_B"=w622, "PING_C"=w622, "PING_D"=w622) -> (w629:T12)
            n62 = Bundle By Name(cluster=w626, "xDistance"=w624, "yDistance"=w624, "wDistance"=w624) -> (w625:T13)
          }
          frame "ARDUINO MODE 0" {
          }
          frame "ARDUINO MODE 1" {
          }
          frame "NAVX CALIBRATE" {
            # "Adds a 15 second delay to the startup process \nfor the NavX to calibrate"
            n63 = Wait (ms)(milliseconds to wait=u32 5000) -> ()  [unwired: 1 out]
          }
          frame "NO ACTION", Default {
            n64 = case shown="4" w649 {
              tunnel: [0 100] -> w651
              frame 1, Default {
              }
              frame 4 {
              }
            }
          }
          frame "----RESET CASES----" {
          }
          frame "RESET ENCODERS" {
          }
          frame "RESET FLAGS" {
            w665 = 0
            # "Resets any software variables\nand/or non-critical states"
            n65 = Wait (ms)(milliseconds to wait=u32 20) -> ()  [unwired: 1 out]
            n66 = Bundle By Name(cluster=w669, "PING_A"=w665, "PING_B"=w665, "PING_C"=w665, "PING_D"=w665) -> (w668:T12)
          }
          frame "RESET YAW" {
            n67 = Wait (ms)(milliseconds to wait=u32 100) -> ()  [unwired: 1 out]
          }
        }
        "State Logic" <- w145
        n68 = call "navX reading VI.vi"("Mode"=w130) -> ("NavX Readings"=w131:T4, "Status"=→"Status":T3)  [unwired: 2 in, 2 out]
        "NavX Readings" <- w131
        n69 = Unbundle By Name(w131) -> ("Yaw"=w129:dbl)
        n70 = local write "Arduino Mode"(w136) -> ()
        n71 = local read "TASK ENABLE"() -> (w135:bool)
        n72 = call "Motor Control NO PID.vi"("Yaw"=w129, "Speed"=w139, "Direction"=w137) -> ("Speed & distance"=→"Speed & distance":T7)  [unwired: 1 in, 1 out]
        n73 = Not(x=w135) -> (.not. x?=w134:bool)
        n74 = case shown="True" w146 {
          tunnel: w150 -> [w168 w185]
          tunnel: w154 -> [w164 w187]
          tunnel: [w168 w185] -> w159
          tunnel: [w164 w188] -> w158
          tunnel: w155 -> [_ w183]
          tunnel: w157 -> [_ w184]
          tunnel: w152 -> [w167 w190]
          tunnel: [w167 w190] -> w151
          tunnel: "STOP TASK" -> [_ w173]
          tunnel: w145 -> [w166 w189]
          tunnel: [w166 w186] -> w144
          tunnel: w141 -> [w165 w179]
          tunnel: [w165 w179] -> w140
          tunnel: w134 -> [_ w174]
          tunnel: [w163 w171] -> w133
          tunnel: w132 -> [w163 w170]
          tunnel: [_ w169] -> w127
          frame False {
          }
          frame True {
            # ">>Action Queue>>"
            # ">>State Logic Queue Reference >>"
            n75 = Or(x=w173, y=w174) -> (x .or. y?=w172:bool)
            n76 = Unbundle By Name(w179) -> ("xDistance"=w176:dbl, "yDistance"=w177:dbl, "wDistance"=w178:dbl)
            n77 = Unbundle By Name(w190) -> ("PING_A"=w182:u8, "PING_B"=w181:u8, "PING_C"=w180:u8, "PING_D"=w175:u8)
            n78 = case shown="11" w189 {
              tunnel: [w192 w195 w206 w214 w259 w271 w307 w353 w397 w454 w491] -> w188
              tunnel: w187 -> [w192 w198 w207 w217 w261 w272 w308 w354 w403 w447 w495]
              tunnel: [State_Type_Definitions,_for_0.26g_versions_and_later_2."Idle" ("Enum") State_Type_Definitions,_for_0.26g_versions_and_later_2."Idle" ("Enum") w202 w216 State_Type_Definitions,_for_0.26g_versions_and_later_2."Shutdown" ("Enum") w273 w310 w352 w398 w453 w492] -> w186
              tunnel: w185 -> [_ _ w205 w220 _ w278 w320 w361 w402 w451 w496]
              tunnel: w184 -> [_ _ _ w219 _ w277 w319 w360 w401 w450 w488]
              tunnel: w183 -> [_ _ w204 w215 _ w276 w318 w359 w400 w449 w487]
              tunnel: w172 -> [_ _ _ _ _ w270 w309 w356 w396 w452 w493]
              tunnel: w182 -> [_ _ _ _ _ _ _ _ _ _ _]
              tunnel: w181 -> [_ _ _ _ _ _ w316 _ w394 w442 w498]
              tunnel: w180 -> [_ _ _ _ _ _ w315 _ w395 w443 w497]
              tunnel: w178 -> [_ _ _ _ _ _ _ w358 _ _ _]
              tunnel: w177 -> [_ _ _ _ _ w269 _ _ _ _ _]
              tunnel: w176 -> [_ _ _ _ _ _ _ _ _ w438 _]
              tunnel: w175 -> [_ _ _ _ _ _ _ _ _ _ _]
              tunnel: [State_Type_Definitions,_for_0.26g_versions_and_later_2."Idle" ("Enum") State_Type_Definitions,_for_0.26g_versions_and_later_2."Idle" ("Enum") State_Type_Definitions,_for_0.26g_versions_and_later_2."Idle" ("Enum") State_Type_Definitions,_for_0.26g_versions_and_later_2."Idle" ("Enum") State_Type_Definitions,_for_0.26g_versions_and_later_2."Shutdown" ("Enum") w266 w306 w349 w389 w437 w490] -> w171
              tunnel: w170 -> [_ _ w202 _ _ _ _ _ _ _ _]
              tunnel: [_ _ _ TRUE ("Green LED") _ _ _ _ _ _ _] -> w169
              frame 0 {
              }
              frame 1 {
                n79 = for {
                  shift-right: [w201] -> w195
                  shift-left: w198 -> [w200]
                  tunnel: string[] ["INIT", "NAVX CALIBRATE", "RESET FLAGS", "RESET YAW", "ARDUINO MODE 0"] -> [w199] mode=indexing
                  n80 = Enqueue Element(queue=w200, element=w199) -> (queue out=w201:refnum<queue>)  [unwired: 2 in, 2 out]
                }
              }
              frame 3 {
                n81 = Flush Queue(queue=w205, error in (no error)=w204) -> ()  [unwired: 3 out]
                n82 = for {
                  shift-right: [w211] -> w206
                  shift-left: w207 -> [w210]
                  tunnel: string[] ["STOP", "RESET ENCODERS", "RESET YAW", "ARDUINO MODE 0"] -> [w209] mode=indexing
                  n83 = Enqueue Element(queue=w210, element=w209) -> (queue out=w211:refnum<queue>)  [unwired: 2 in, 2 out]
                }
              }
              frame 4, Default {
                n84 = Dequeue Element(queue=w220, timeout in ms (-1)=w219, error in (no error)=w215) -> (element=w218:T9)  [unwired: 3 out]
                n85 = case shown="\"Start Task 4\"" w218 {
                  tunnel: [w222 w229 w236 w243 w250 w252] -> w214
                  tunnel: w217 -> [w223 w230 w237 w244 w250 w253]
                  tunnel: [State_Type_Definitions."Task 1" ("Enum") State_Type_Definitions."Task 2" ("Enum") State_Type_Definitions,_for_0.26g_versions_and_later_2."Task 3" ("Enum") State_Type_Definitions,_for_0.26g_versions_and_later_2."Task 4_A" ("Enum") State_Type_Definitions,_for_0.26g_versions_and_later_2."Idle" ("Enum") State_Type_Definitions,_for_0.26g_versions_and_later_2."Shutdown" ("Enum")] -> w216
                  frame "Start Task 1" {
                    n86 = for {
                      shift-right: [w227] -> w222
                      shift-left: w223 -> [w226]
                      tunnel: string[] ["RESET ENCODERS", "RESET YAW", "FORWARD", "READ ENCODERS"] -> [w225] mode=indexing
                      n87 = Enqueue Element(queue=w226, element=w225) -> (queue out=w227:refnum<queue>)  [unwired: 2 in, 2 out]
                    }
                  }
                  frame "Start Task 2" {
                    n88 = for {
                      shift-right: [w234] -> w229
                      shift-left: w230 -> [w233]
                      tunnel: string[] ["RESET ENCODERS", "RESET YAW", "ULTRASONIC READ", "ARDUINO MODE 0"] -> [w232] mode=indexing
                      n89 = Enqueue Element(queue=w233, element=w232) -> (queue out=w234:refnum<queue>)  [unwired: 2 in, 2 out]
                    }
                  }
                  frame "Start Task 3" {
                    n90 = for {
                      shift-right: [w241] -> w236
                      shift-left: w237 -> [w240]
                      tunnel: string[] ["RESET ENCODERS", "READ ENCODERS", "R-ACW"] -> [w239] mode=indexing
                      n91 = Enqueue Element(queue=w240, element=w239) -> (queue out=w241:refnum<queue>)  [unwired: 2 in, 2 out]
                    }
                  }
                  frame "Start Task 4" {
                    n92 = for {
                      shift-right: [w248] -> w243
                      shift-left: w244 -> [w247]
                      tunnel: string[] ["STOP", "RESET YAW", "RESET ENCODERS", "ARDUINO MODE 0", "ULTRASONIC READ", "FORWARD"] -> [w246] mode=indexing
                      n93 = Enqueue Element(queue=w247, element=w246) -> (queue out=w248:refnum<queue>)  [unwired: 2 in, 2 out]
                    }
                  }
                  frame "None", Default {
                  }
                  frame "Exit" {
                    n94 = for {
                      shift-right: [w257] -> w252
                      shift-left: w253 -> [w256]
                      tunnel: string[] ["STOP", "RESET ENCODERS", "RESET YAW", "EXIT"] -> [w255] mode=indexing
                      n95 = Enqueue Element(queue=w256, element=w255) -> (queue out=w257:refnum<queue>)  [unwired: 2 in, 2 out]
                    }
                  }
                }
              }
              frame 5 {
                n96 = for {
                  shift-right: [w265] -> w259
                  shift-left: w261 -> [w264]
                  tunnel: string[] ["INIT", "RESET ENCODERS", "RESET FLAGS", "EXIT"] -> [w263] mode=indexing
                  n97 = Enqueue Element(queue=w264, element=w263) -> (queue out=w265:refnum<queue>)  [unwired: 2 in, 2 out]
                }
              }
              frame 6 {
                # "Use 250"
                n98 = Dequeue Element(queue=w278, timeout in ms (-1)=w277, error in (no error)=w276) -> (element=w275:T9)  [unwired: 3 out]
                n99 = Greater?(x=w269, y=10000.0) -> (0:w267:bool)
                n100 = Or(x=w267, y=w270) -> (x .or. y?=w274:bool)
                n101 = case shown="\"None\", Default" w275 {
                  tunnel: w274 -> [w281 _]
                  tunnel: [w285 State_Type_Definitions,_for_0.26g_versions_and_later_2."True Stop" ("Enum")] -> w273
                  tunnel: w272 -> [w282 w300]
                  tunnel: [w280 w299] -> w271
                  tunnel: [State_Type_Definitions,_for_0.26g_versions_and_later_2."Idle" ("Enum") State_Type_Definitions,_for_0.26g_versions_and_later_2."Shutdown" ("Enum")] -> w266
                  frame "None", Default {
                    n102 = case shown="True" w281 {
                      tunnel: w282 -> [w288 w294]
                      tunnel: [w287 w292] -> w280
                      frame False {
                        n103 = for {
                          shift-right: [w290] -> w287
                          shift-left: w288 -> [w291]
                          tunnel: string[] ["READ ENCODERS", "FORWARD"] ("element") -> [w289] mode=indexing
                          n104 = Enqueue Element(queue=w291, element=w289) -> (queue out=w290:refnum<queue>)  [unwired: 2 in, 2 out]
                        }
                      }
                      frame True {
                        n105 = for {
                          shift-right: [w296] -> w292
                          shift-left: w294 -> [w297]
                          tunnel: string[] ["RESET YAW", "RESET ENCODERS", "STOP", "ARDUINO MODE 0"] -> [w295] mode=indexing
                          n106 = Enqueue Element(queue=w297, element=w295) -> (queue out=w296:refnum<queue>)  [unwired: 2 in, 2 out]
                        }
                      }
                    }
                    n107 = Select(t=State_Type_Definitions,_for_0.26g_versions_and_later_2."True Stop" ("Enum"), s=w281, f=State_Type_Definitions."Task 1" ("Enum")) -> (s? t:f=w285:u16)
                  }
                  frame "Exit" {
                    n108 = for {
                      shift-right: [w304] -> w299
                      shift-left: w300 -> [w305]
                      tunnel: string[] ["STOP", "RESET ENCODERS", "RESET YAW", ""] -> [w303] mode=indexing
                      n109 = Enqueue Element(queue=w305, element=w303) -> (queue out=w304:refnum<queue>)  [unwired: 2 in, 2 out]
                    }
                  }
                }
              }
              frame 7 {
                w314 = u16 20 ("y")
                # ">>Object detected>>"
                n110 = Dequeue Element(queue=w320, timeout in ms (-1)=w319, error in (no error)=w318) -> (element=w317:T9)  [unwired: 3 out]
                n111 = Less?(x=w316, y=w314) -> (x < y?=w313:bool)
                n112 = Less?(x=w315, y=w314) -> (x < y?=w312:bool)
                n113 = Or(x=w313, y=w312) -> (x .or. y?=w311:bool)
                "Object detected?" <- w311
                n114 = case shown="\"Exit\"" w317 {
                  tunnel: w311 -> [w324 _]
                  tunnel: [w326 State_Type_Definitions,_for_0.26g_versions_and_later_2."True Stop" ("Enum")] -> w310
                  tunnel: w309 -> [w325 _]
                  tunnel: w308 -> [w323 w343]
                  tunnel: [w322 w344] -> w307
                  tunnel: [State_Type_Definitions,_for_0.26g_versions_and_later_2."Idle" ("Enum") State_Type_Definitions,_for_0.26g_versions_and_later_2."Shutdown" ("Enum")] -> w306
                  frame "None", Default {
                    n115 = case shown="True" w324 {
                      tunnel: w323 -> [w330 w337]
                      tunnel: [w331 w336] -> w322
                      frame False {
                        n116 = for {
                          tunnel: string[] ["ULTRASONIC READ", "STOP"] ("element") -> [w332] mode=indexing
                          shift-right: [w334] -> w331
                          shift-left: w330 -> [w333]
                          n117 = Enqueue Element(queue=w333, element=w332) -> (queue out=w334:refnum<queue>)  [unwired: 2 in, 2 out]
                        }
                      }
                      frame True {
                        n118 = for {
                          shift-right: [w339] -> w336
                          shift-left: w337 -> [w340]
                          tunnel: string[] ["REVERSE", "ULTRASONIC READ"] -> [w338] mode=indexing
                          n119 = Enqueue Element(queue=w340, element=w338) -> (queue out=w339:refnum<queue>)  [unwired: 2 in, 2 out]
                        }
                      }
                    }
                    n120 = Select(t=State_Type_Definitions,_for_0.26g_versions_and_later_2."True Stop" ("Enum"), s=w325, f=State_Type_Definitions."Task 2" ("Enum")) -> (s? t:f=w326:u16)
                  }
                  frame "Exit" {
                    n121 = for {
                      shift-right: [w347] -> w344
                      shift-left: w343 -> [w348]
                      tunnel: string[] ["STOP", "RESET ENCODERS", "RESET YAW", "ARDUINO MODE 0"] -> [w346] mode=indexing
                      n122 = Enqueue Element(queue=w348, element=w346) -> (queue out=w347:refnum<queue>)  [unwired: 2 in, 2 out]
                    }
                  }
                }
              }
              frame 10 {
                n123 = Dequeue Element(queue=w361, timeout in ms (-1)=w360, error in (no error)=w359) -> (element=w350:T9)  [unwired: 3 out]
                n124 = Greater?(x=w358, y=150.0) -> (0:w355:bool)
                n125 = Or(x=w355, y=w356) -> (x .or. y?=w351:bool)
                n126 = case shown="\"Exit\"" w350 {
                  tunnel: w351 -> [w364 _]
                  tunnel: [w368 State_Type_Definitions,_for_0.26g_versions_and_later_2."True Stop" ("Enum")] -> w352
                  tunnel: w354 -> [w365 w384]
                  tunnel: [w363 w383] -> w353
                  tunnel: [State_Type_Definitions,_for_0.26g_versions_and_later_2."Idle" ("Enum") State_Type_Definitions,_for_0.26g_versions_and_later_2."Shutdown" ("Enum")] -> w349
                  frame "None", Default {
                    n127 = case shown="False" w364 {
                      tunnel: w365 -> [w371 w377]
                      tunnel: [w370 w375] -> w363
                      frame False {
                        n128 = for {
                          shift-right: [w373] -> w370
                          shift-left: w371 -> [w374]
                          tunnel: string[] ["READ ENCODERS", "R-ACW"] ("element") -> [w372] mode=indexing
                          n129 = Enqueue Element(queue=w374, element=w372) -> (queue out=w373:refnum<queue>)  [unwired: 2 in, 2 out]
                        }
                      }
                      frame True {
                        n130 = for {
                          shift-right: [w379] -> w375
                          shift-left: w377 -> [w380]
                          tunnel: string[] ["RESET YAW", "RESET ENCODERS", "STOP", "ARDUINO MODE 0"] -> [w378] mode=indexing
                          n131 = Enqueue Element(queue=w380, element=w378) -> (queue out=w379:refnum<queue>)  [unwired: 2 in, 2 out]
                        }
                      }
                    }
                    n132 = Select(t=State_Type_Definitions,_for_0.26g_versions_and_later_2."True Stop" ("Enum"), s=w364, f=State_Type_Definitions,_for_0.26g_versions_and_later_2."Task 3" ("Enum")) -> (s? t:f=w368:T8)
                  }
                  frame "Exit" {
                    n133 = for {
                      shift-right: [w387] -> w383
                      shift-left: w384 -> [w388]
                      tunnel: string[] ["STOP", "RESET ENCODERS", "RESET YAW", ""] -> [w386] mode=indexing
                      n134 = Enqueue Element(queue=w388, element=w386) -> (queue out=w387:refnum<queue>)  [unwired: 2 in, 2 out]
                    }
                  }
                }
              }
              frame 11 {
                w393 = 50
                # ">> Outputs true if object detected >>"
                # ">> Manual override >>"
                n135 = Dequeue Element(queue=w402, timeout in ms (-1)=w401, error in (no error)=w400) -> (element=w399:T9)  [unwired: 3 out]
                n136 = Less?(x=w395, y=w393) -> (x < y?=w391:bool)
                n137 = Less?(x=w394, y=w393) -> (x < y?=w392:bool)
                n138 = And(x=w392, y=w391) -> (x .and. y?=w390:bool)
                "Detect?" <- w390
                n139 = case shown="\"None\", Default" w399 {
                  tunnel: [w412 State_Type_Definitions,_for_0.26g_versions_and_later_2."True Stop" ("Enum")] -> w398
                  tunnel: [w410 w431] -> w397
                  tunnel: w403 -> [w409 _]
                  tunnel: w396 -> [w407 _]
                  tunnel: w390 -> [w405 _]
                  tunnel: [w404 State_Type_Definitions,_for_0.26g_versions_and_later_2."Shutdown" ("Enum")] -> w389
                  frame "None", Default {
                    # ">> WIill proceed to part ii if not manual override >>"
                    # ">>If ENABLE or Trigger is set to true>>"
                    n140 = Or(x=w405, y=w407) -> (x .or. y?=w406:bool)
                    n141 = case shown="False" w406 {
                      tunnel: [w419 w424] -> w410
                      tunnel: w409 -> [w417 w423]
                      frame False {
                        n142 = for {
                          shift-right: [w421] -> w419
                          shift-left: w417 -> [w422]
                          tunnel: string[] ["FORWARD", "ULTRASONIC READ", ""] ("element") -> [w420] mode=indexing
                          n143 = Enqueue Element(queue=w422, element=w420) -> (queue out=w421:refnum<queue>)  [unwired: 2 in, 2 out]
                        }
                      }
                      frame True {
                        n144 = for {
                          shift-right: [w427] -> w424
                          shift-left: w423 -> [w428]
                          tunnel: string[] ["STOP", "RESET ENCODERS", "RESET YAW", "ARDUINO MODE 0"] -> [w426] mode=indexing
                          n145 = Enqueue Element(queue=w428, element=w426) -> (queue out=w427:refnum<queue>)  [unwired: 2 in, 2 out]
                        }
                      }
                    }
                    n146 = case shown="True" w407 {
                      tunnel: [State_Type_Definitions,_for_0.26g_versions_and_later_2."True Stop" ("Enum") State_Type_Definitions,_for_0.26g_versions_and_later_2."True Stop" ("Enum")] -> w408
                      tunnel: [State_Type_Definitions,_for_0.26g_versions_and_later_2."Task 4_B" ("Enum") State_Type_Definitions,_for_0.26g_versions_and_later_2."Idle" ("Enum")] -> w404
                      frame False {
                      }
                      frame True {
                      }
                    }
                    n147 = Select(t=w408, s=w406, f=State_Type_Definitions,_for_0.26g_versions_and_later_2."Task 4_A" ("Enum")) -> (s? t:f=w412:T8)
                  }
                  frame "Exit" {
                    n148 = for {
                      shift-right: [w434] -> w431
                      shift-left: _ -> [w435]
                      tunnel: string[] ["STOP", "RESET ENCODERS", "RESET YAW", ""] -> [w433] mode=indexing
                      n149 = Enqueue Element(queue=w435, element=w433) -> (queue out=w434:refnum<queue>)  [unwired: 2 in, 2 out]
                    }
                  }
                }
              }
              frame 12 {
                w446 = 20
                # ">> Outputs true if 150 mm has been moved >>"
                # ">> Outputs true if sensor not obstructed>>"
                # ">> Manual override >>"
                n150 = Dequeue Element(queue=w451, timeout in ms (-1)=w450, error in (no error)=w449) -> (element=w448:T9)  [unwired: 3 out]
                n151 = Greater?(x=w443, y=w446) -> (0:w444:bool)
                n152 = Greater?(x=w442, y=w446) -> (0:w445:bool)
                n153 = Greater Or Equal?(x=w438, y=80.0) -> (x >= y?=w440:bool)
                n154 = And(x=w445, y=w444) -> (x .and. y?=w439:bool)
                n155 = And(x=w440, y=w439) -> (x .and. y?=w436:bool)
                n156 = case shown="\"None\", Default" w448 {
                  tunnel: [w463 State_Type_Definitions,_for_0.26g_versions_and_later_2."True Stop" ("Enum")] -> w453
                  tunnel: [w461 w482] -> w454
                  tunnel: w447 -> [w460 _]
                  tunnel: w452 -> [w458 _]
                  tunnel: w436 -> [w456 _]
                  tunnel: [w455 State_Type_Definitions,_for_0.26g_versions_and_later_2."Shutdown" ("Enum")] -> w437
                  frame "None", Default {
                    # ">> WIill proceed to part ii if not manual override >>"
                    # ">>If ENABLE or Trigger is set to true>>"
                    n157 = Or(x=w456, y=w458) -> (x .or. y?=w457:bool)
                    n158 = case shown="False" w457 {
                      tunnel: [w470 w475] -> w461
                      tunnel: w460 -> [w468 w474]
                      frame False {
                        n159 = for {
                          shift-right: [w472] -> w470
                          shift-left: w468 -> [w473]
                          tunnel: string[] ["RIGHT", "ULTRASONIC READ", "READ ENCODERS"] ("element") -> [w471] mode=indexing
                          n160 = Enqueue Element(queue=w473, element=w471) -> (queue out=w472:refnum<queue>)  [unwired: 2 in, 2 out]
                        }
                      }
                      frame True {
                        n161 = for {
                          shift-right: [w478] -> w475
                          shift-left: w474 -> [w479]
                          tunnel: string[] ["STOP", "RESET ENCODERS", "RESET YAW", "ARDUINO MODE 0"] -> [w477] mode=indexing
                          n162 = Enqueue Element(queue=w479, element=w477) -> (queue out=w478:refnum<queue>)  [unwired: 2 in, 2 out]
                        }
                      }
                    }
                    n163 = case shown="False" w458 {
                      tunnel: [State_Type_Definitions,_for_0.26g_versions_and_later_2."True Stop" ("Enum") State_Type_Definitions,_for_0.26g_versions_and_later_2."True Stop" ("Enum")] -> w459
                      tunnel: [State_Type_Definitions,_for_0.26g_versions_and_later_2."Task 4_C" ("Enum") State_Type_Definitions,_for_0.26g_versions_and_later_2."Idle" ("Enum")] -> w455
                      frame False {
                      }
                      frame True {
                      }
                    }
                    n164 = Select(t=w459, s=w457, f=State_Type_Definitions,_for_0.26g_versions_and_later_2."Task 4_B" ("Enum")) -> (s? t:f=w463:T8)
                  }
                  frame "Exit" {
                    n165 = for {
                      shift-right: [w485] -> w482
                      shift-left: _ -> [w486]
                      tunnel: string[] ["STOP", "RESET ENCODERS", "RESET YAW", ""] -> [w484] mode=indexing
                      n166 = Enqueue Element(queue=w486, element=w484) -> (queue out=w485:refnum<queue>)  [unwired: 2 in, 2 out]
                    }
                  }
                }
              }
              frame 13 {
                w501 = 30
                # ">> Outputs true if object detected >>"
                # ">> Manual override >>"
                n167 = Dequeue Element(queue=w496, timeout in ms (-1)=w488, error in (no error)=w487) -> (element=w489:T9)  [unwired: 3 out]
                n168 = Less?(x=w497, y=w501) -> (x < y?=w499:bool)
                n169 = Less?(x=w498, y=w501) -> (x < y?=w500:bool)
                n170 = And(x=w500, y=w499) -> (x .and. y?=w494:bool)
                n171 = case shown="\"None\", Default" w489 {
                  tunnel: [w510 State_Type_Definitions,_for_0.26g_versions_and_later_2."True Stop" ("Enum")] -> w492
                  tunnel: [w508 w530] -> w491
                  tunnel: w495 -> [w507 w527]
                  tunnel: w493 -> [w505 _]
                  tunnel: w494 -> [w503 _]
                  tunnel: [w502 State_Type_Definitions,_for_0.26g_versions_and_later_2."Shutdown" ("Enum")] -> w490
                  frame "None", Default {
                    # ">> WIill proceed to part ii if not manual override >>"
                    # ">>If ENABLE or Trigger is set to true>>"
                    n172 = Or(x=w503, y=w505) -> (x .or. y?=w504:bool)
                    n173 = case shown="False" w504 {
                      tunnel: [w517 w522] -> w508
                      tunnel: w507 -> [w515 w521]
                      frame False {
                        n174 = for {
                          shift-right: [w519] -> w517
                          shift-left: w515 -> [w520]
                          tunnel: string[] ["FORWARD", "ULTRASONIC READ", ""] ("element") -> [w518] mode=indexing
                          n175 = Enqueue Element(queue=w520, element=w518) -> (queue out=w519:refnum<queue>)  [unwired: 2 in, 2 out]
                        }
                      }
                      frame True {
                        n176 = for {
                          shift-right: [w525] -> w522
                          shift-left: w521 -> [w526]
                          tunnel: string[] ["STOP", "RESET ENCODERS", "RESET YAW", "ARDUINO MODE 0"] -> [w524] mode=indexing
                          n177 = Enqueue Element(queue=w526, element=w524) -> (queue out=w525:refnum<queue>)  [unwired: 2 in, 2 out]
                        }
                      }
                    }
                    n178 = case shown="True" w505 {
                      tunnel: [State_Type_Definitions,_for_0.26g_versions_and_later_2."True Stop" ("Enum") State_Type_Definitions,_for_0.26g_versions_and_later_2."True Stop" ("Enum")] -> w506
                      tunnel: [State_Type_Definitions,_for_0.26g_versions_and_later_2."Idle" ("Enum") State_Type_Definitions,_for_0.26g_versions_and_later_2."Idle" ("Enum")] -> w502
                      frame False {
                      }
                      frame True {
                      }
                    }
                    n179 = Select(t=w506, s=w504, f=State_Type_Definitions,_for_0.26g_versions_and_later_2."Task 4_C" ("Enum")) -> (s? t:f=w510:T8)
                  }
                  frame "Exit" {
                    n180 = for {
                      shift-right: [w533] -> w530
                      shift-left: w527 -> [w534]
                      tunnel: string[] ["STOP", "RESET ENCODERS", "RESET YAW", ""] -> [w532] mode=indexing
                      n181 = Enqueue Element(queue=w534, element=w532) -> (queue out=w533:refnum<queue>)  [unwired: 2 in, 2 out]
                    }
                  }
                }
              }
            }
          }
        }
        n182 = local write "Green LED"(w127) -> ()
      }
      n183 = call <vilib>:"DIO Close.vi"("error in (no error)"=w7, "DIO Info In"=w10) -> ()  [unwired: 9 in, 1 out]
      n184 = call <vilib>:"DIO Close.vi"("error in (no error)"=w17, "DIO Info In"=w19) -> ()  [unwired: 9 in, 1 out]
      n185 = call <vilib>:"NavX Close.vi"("error in (no error)"=w5, "NavX Info In"=w6) -> ()  [unwired: 9 in, 1 out]
      n186 = call <vilib>:"DIO Close.vi"("error in (no error)"=w12, "DIO Info In"=w14) -> ()  [unwired: 9 in, 1 out]
      n187 = Merge Errors "Merge Errors"(w47, w46) -> (w29:errorcluster)
      n188 = Merge Errors(w33, w29) -> (w28:errorcluster)
      n189 = Destroy User Event(user event=w50, error in=w28) -> ()  [unwired: 1 out]
      n190 = Destroy User Event(user event=w51, error in=w28) -> ()  [unwired: 1 out]
      n191 = Unregister For Events(event registration refnum=w42, error in=w28) -> ()  [unwired: 1 out]
      n192 = Release Queue(queue=w24, error in (no error)=w28) -> (error out=w4:errorcluster)  [unwired: 1 in, 2 out]
      n193 = Release Queue(queue=w41, error in (no error)=w28) -> ()  [unwired: 1 in, 3 out]
      n194 = call <vilib>:"Simple Error Handler.vi"("error in (no error)"=w4) -> ("error out"=w3:errorcluster)  [unwired: 4 in, 4 out]
      n195 = call <vilib>:"Reset myRIO.vi"("error in (no error)"=w3) -> ("error out"=→"error out":errorcluster)  [unwired: 10 in]
    }
    frame #2 {
      n196 = Wait (ms)(milliseconds to wait=u32 100) -> ()  [unwired: 1 out]
    }
  }
